vi "createILCADC.vi"(8 "error in (no error)":errorcluster, 10 "Channel":u8, 11 "ILCADCFactory in":refnum<class "ILCADCFactory.lvclass">) -> (0 "error out":errorcluster, 2 "ILCADC":refnum<class "IILCADC.lvclass">, 3 "ILCADCFactory out":refnum<class "ILCADCFactory.lvclass">)   [LabVIEW 2015, in "ILCADCFactory.lvclass"]
uses:
  ILCADCFactory.lvclass
  ILCADC/IILCADC/IILCADC.lvclass
  ILCADC/ILCADC1/ILCADC1.lvclass
  ILCADC/ILCADC2/ILCADC2.lvclass
  ILCADC/ILCADC3/ILCADC3.lvclass
  ILCADC/ILCADC4/ILCADC4.lvclass
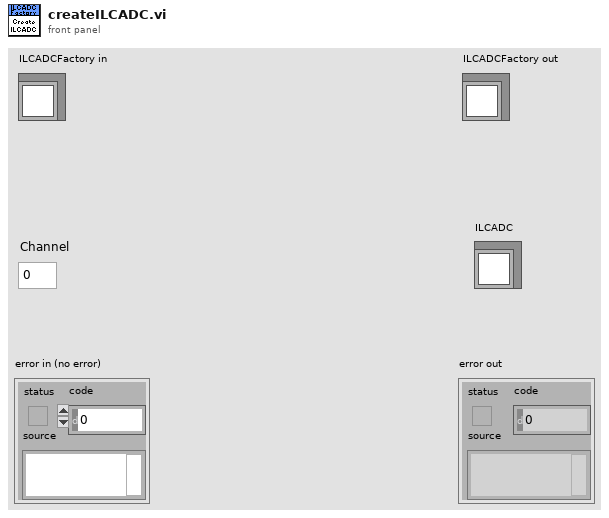
[diagram p1: front panel]
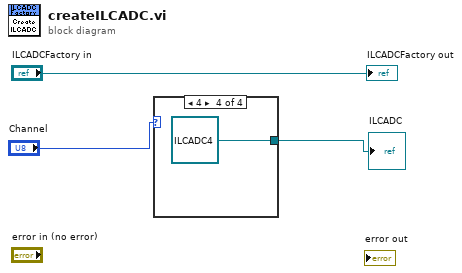
[diagram p0: block diagram]
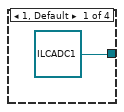
[diagram p2: hidden frame]
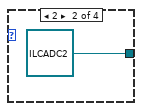
[diagram p3: hidden frame]
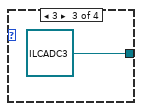
[diagram p4: hidden frame]
diagram:
  n1 = case shown="4" "Channel" {
    tunnel: [refnum<class "ILCADC1.lvclass"> refnum ("ILCADC1.lvclass") refnum<class "ILCADC2.lvclass"> refnum ("ILCADC2.lvclass") refnum<class "ILCADC3.lvclass"> refnum ("ILCADC3.lvclass") refnum<class "ILCADC4.lvclass"> refnum ("ILCADC4.lvclass")] -> w1
    frame 1, Default {
    }
    frame 2 {
    }
    frame 3 {
    }
    frame 4 {
    }
  }
  "ILCADC" <- w1
  "ILCADCFactory out" <- "ILCADCFactory in"
